vi "GetWaveformAssetId.vi"(11 "waveform in":waveform(sgl)) -> (2 "asset id":string, 3 "waveform out":waveform(sgl))   [LabVIEW 2017]
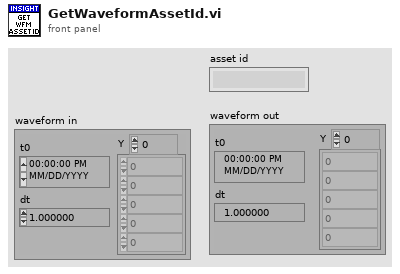
[diagram p1: front panel]
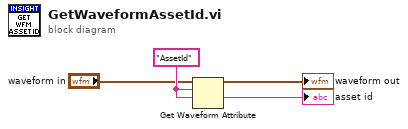
[diagram p0: block diagram]
diagram:
  w2 = "AssetId" ("name")
  n1 = Get Waveform Attribute(5:w2, 6:w2, 7:"waveform in") -> (1:→"asset id":string, 3:→"waveform out":waveform(sgl))  [unwired: 1 in, 2 out]
